vi "IND560 Stable Weigth Gross Equal Net.vi"(8 "Error In":errorcluster, 11 "read buffer":string) -> (0 "Error Out":errorcluster, 1 "IND560 Selector":T1, 3 "Gross and Net Weight":dbl)   [LabVIEW 2016]
uses:
  Type Definitions/IND560 Data Output Selector.ctl
panel:
  out "x .xor. y?":bool
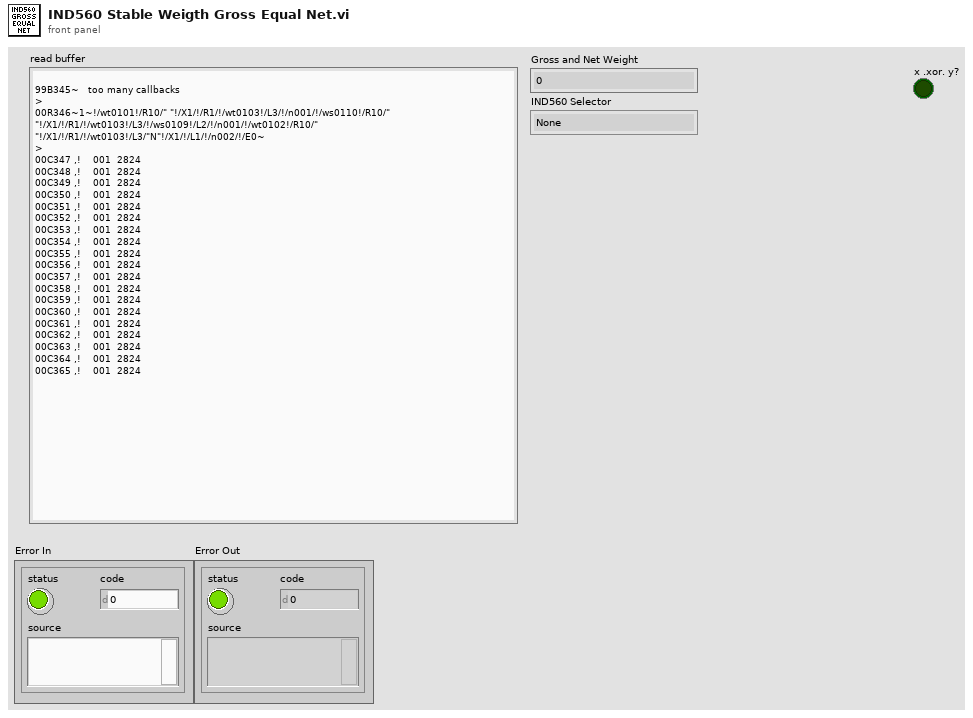
[diagram p1: front panel]
types:
  T1 = typedef "IND560 Data Output Selector.ctl" = enum16{"None", "Use Gross Not Equal Net", "Use Gross Equal Net", "Use Unstable Weights"}
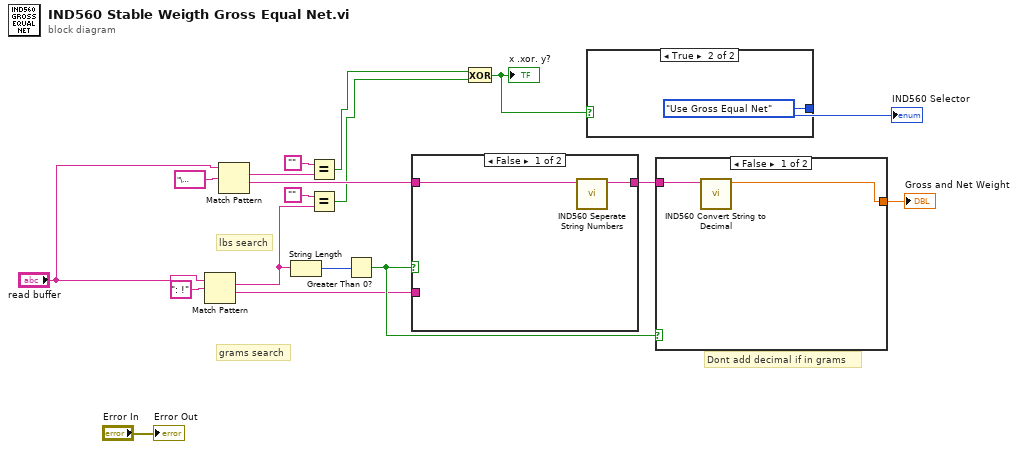
[diagram p0: block diagram]
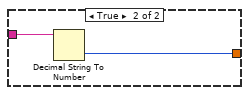
[diagram p2: hidden frame]
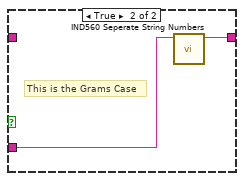
[diagram p3: hidden frame]
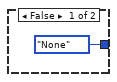
[diagram p4: hidden frame]
diagram:
  # "Dont add decimal if in grams"
  # "grams search"
  # "lbs search"
  n1 = Match Pattern(string="read buffer", regular expression=": !") -> (match substring=w7:string, after substring=w5:string)  [unwired: 1 in, 2 out]
  n2 = Match Pattern(string="read buffer", regular expression="\u0002,    ") -> (match substring=w16:string, after substring=w9:string)  [unwired: 1 in, 2 out]
  n3 = String Length(string=w7) -> (length=w8:i32)
  n4 = Equal?(x="", y=w16) -> (x = y?=w3:bool)
  n5 = Equal?(x="", y=w7) -> (x = y?=w2:bool)
  n6 = Greater Than 0?(x=w8) -> (x > 0?=w6:bool)
  n7 = case shown="False" w6 {
    tunnel: w9 -> [w20 _]
    tunnel: [w19 w21] -> w12
    tunnel: w5 -> [_ w22]
    frame False {
      n8 = call "IND560 Seperate String Numbers.vi"("read buffer"=w20) -> ("Net Weight"=w19:string)  [unwired: 9 in, 1 out]
    }
    frame True {
      # "This is the Grams Case"
      n9 = call "IND560 Seperate String Numbers.vi"("read buffer"=w22) -> ("Net Weight"=w21:string)  [unwired: 9 in, 1 out]
    }
  }
  n10 = Exclusive Or(1:w2, 2:w3) -> (0:w1:bool)
  "x .xor. y?" <- w1
  n11 = case shown="True" w1 {
    tunnel: [IND560_Data_Output_Selector."None" ("IND560 Selector") IND560_Data_Output_Selector."Use Gross Equal Net" ("IND560 Selector")] -> w14
    frame False {
    }
    frame True {
    }
  }
  "IND560 Selector" <- w14
  n12 = case shown="False" w6 {
    tunnel: [w26 w27] -> w13
    tunnel: w12 -> [w25 w28]
    frame False {
      n13 = call "IND560 Convert String to Decimal.vi"("read buffer"=w25) -> ("Weigth"=w26:dbl)  [unwired: 9 in, 1 out]
    }
    frame True {
      n14 = Decimal String To Number(string=w28) -> (number=w27:i32)  [unwired: 2 in, 1 out]
    }
  }
  "Gross and Net Weight" <- w13
  "Error Out" <- "Error In"
